vi "form ellipse.vi"(6 "alpha":dbl, 7 "samples":i32, 8 "y0":dbl, 9 "x0":dbl, 10 "b":dbl, 11 "a":dbl) -> (2 "Y":dbl[](array[numeric]), 3 "X":dbl[](array[numeric]))   [LabVIEW 2013]
doc: "Ellipse fit data"
uses:
  <vilib>/Analysis/1siggen.llb/Ramp Pattern by Samples.vi
  <vilib>/Analysis/NI_AALBase.lvlib
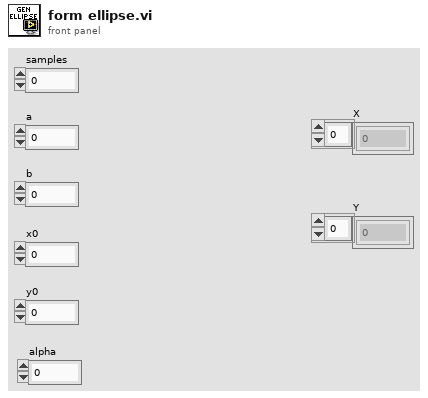
[diagram p1: front panel]
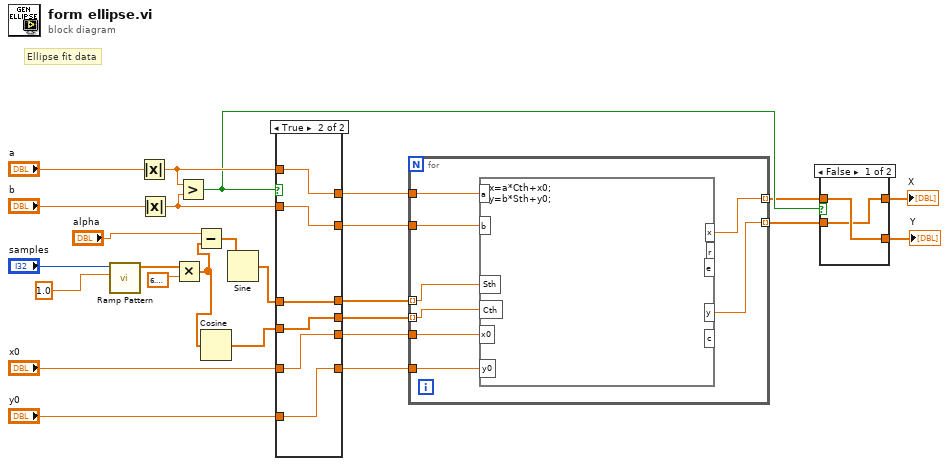
[diagram p0: block diagram]
diagram:
  # "Ellipse fit data"
  n1 = call-poly <vilib>:"Ramp Pattern.vi"("end"=1.0, "samples"="samples") -> ("Ramp Pattern"=w24:dbl[])  [unwired: 8 in, 1 out]
  n2 = Absolute Value(x="a") -> (abs(x)=w21:dbl)
  n3 = Absolute Value(x="b") -> (abs(x)=w20:dbl)
  n4 = Multiply(x=w24, y=6.283185307179586) -> (x*y=w2:dbl[])
  n5 = Greater?(x=w21, y=w20) -> (0:w13:bool)
  n6 = Subtract(x="alpha", y=w2) -> (x-y=w3:dbl[])
  n7 = Cosine(x=w2) -> (cos(x)=w5:dbl[])
  n8 = Sine(x=w3) -> (sin(x)=w4:dbl[])
  n9 = case shown="True" w13 {
    tunnel: w21 -> [w32 w38]
    tunnel: w20 -> [w31 w37]
    tunnel: [w31 w38] -> w19
    tunnel: [w32 w37] -> w18
    tunnel: w4 -> [w30 w36]
    tunnel: w5 -> [w29 w35]
    tunnel: [w29 w36] -> w16
    tunnel: [w30 w35] -> w15
    tunnel: "x0" -> [w28 w34]
    tunnel: "y0" -> [w27 w33]
    tunnel: [w27 w34] -> w7
    tunnel: [w28 w33] -> w6
    frame False {
    }
    frame True {
    }
  }
  n10 = for {
    tunnel: w19 -> [w46]
    tunnel: w18 -> [w45]
    tunnel: w7 -> [w44]
    tunnel: w6 -> [w43]
    tunnel: [w42] -> w12 mode=indexing
    tunnel: [w41] -> w14 mode=indexing
    tunnel: w16 -> [w40] mode=indexing
    tunnel: w15 -> [w39] mode=indexing
    n11 = formula code="x=a*Cth+x0;\ny=b*Sth+y0;"("a"=w46, "b"=w45, "Sth"=w40, "x0"=w44, "y0"=w43, "Cth"=w39) -> ("x"=w42:dbl, "y"=w41:dbl)  [unwired: 3 out]
  }
  n12 = case shown="False" w13 {
    tunnel: w14 -> [w47 w50]
    tunnel: [w48 w50] -> w10
    tunnel: w12 -> [w48 w49]
    tunnel: [w47 w49] -> w11
    frame False {
    }
    frame True {
    }
  }
  "Y" <- w10
  "X" <- w11
